vi "Panther Dashboard for DQMH.vi"   [LabVIEW 2020]
doc: "Start Panther Dashboard for DQMH\n\nScan the project caller for DQMH Modules\nShow the front panel"
uses:
  Panther Dashboard/Panther Dashboard/Panther Dashboard.lvlib
types:
  T1 = enum32{"Invalid", "Standard", "Closed", "Hidden", "Minimized", "Maximized"}
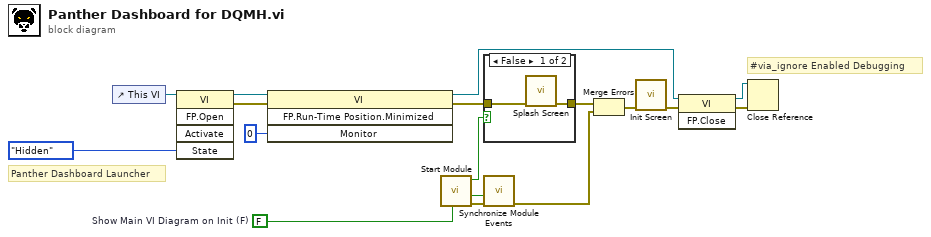
[diagram p0: block diagram]
diagram:
  w8 = FALSE  # Show Main VI Diagram on Init (F)
  # "#via_ignore Enabled Debugging"
  # "Panther Dashboard Launcher"
  n1 = control-ref of="This VI"() -> (w6:refnum<vi>)
  n2 = invoke class="VI" method="FP.Open"(reference=w6, "State"=T1."Hidden") -> (reference out=w3:refnum<vi>, error out=w12:errorcluster)  [unwired: 3 in, 3 out]
  n3 = invoke class="VI" method="FP.Run-Time Position.Minimized"(reference=w3, error in=w12, "Monitor"=i16 0) -> (reference out=w1:refnum<vi>, error out=w15:errorcluster)  [unwired: 1 in, 2 out]
  n4 = call "Start Module.vi"("Show Main VI Diagram on Init (F)"=w8) -> ("error out"=w17:errorcluster, "Wait for Event Sync?"=w9:bool, "Module Was Already Running?"=w4:bool)  [unwired: 6 in, 2 out]
  n5 = case shown="False" w4 {
    tunnel: w15 -> [w19 w20]
    tunnel: [w18 w20] -> w13
    frame False {
      n6 = call "Splash Screen.vi"("error in"=w19) -> ("error out"=w18:errorcluster)  [unwired: 10 in]
    }
    frame True {
    }
  }
  n7 = call "Synchronize Module Events.vi"("error in"=w17, "Wait for Event Sync?"=w9) -> ("error out"=w14:errorcluster)  [unwired: 9 in]
  n8 = Merge Errors(w13, w14) -> (w11:errorcluster)
  n9 = call "Init Screen.vi"("error in"=w11) -> ("error out"=w10:errorcluster)  [unwired: 10 in]
  n10 = invoke class="VI" method="FP.Close"(reference=w1, error in=w10) -> (reference out=w5:refnum<vi>, error out=w16:errorcluster)  [unwired: 1 in, 1 out]
  n11 = Close Reference(reference=w5, error in (no error)=w16) -> ()  [unwired: 1 out]
